vi "LWXPS_GroupMoveAbsolute.vi"(0 "XPS Reference IN":refnum<k24>, 5 "Group Name":string, 7 "Target Position IN":dbl[](array[numeric]), 9 "Number of Positioners":i32, 11 "LabVIEW error IN":errorcluster) -> (4 "XPS Reference OUT":refnum<k24>, 6 "Returned error code":i32, 8 "Target Position OUT":dbl[](array[numeric]), 10 "XPS Error String":string, 15 "LabVIEW error OUT":errorcluster)   [LabVIEW 2020]
uses:
  C:/Users/loasis.BELLANET/Downloads/XPS-UNIFIED/LabVIEW VIs/LabVIEW Source Code/Dll/Newport.XPS.CommandInterface.dll
  Users/loasis.BELLANET/Downloads/XPS-UNIFIED/LabVIEW VIs/LabVIEW Source Code/Dll/Newport.XPS.CommandInterface.dll
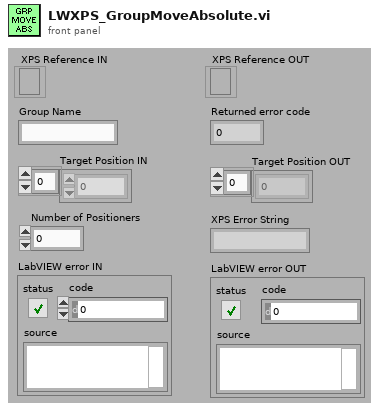
[diagram p1: front panel]
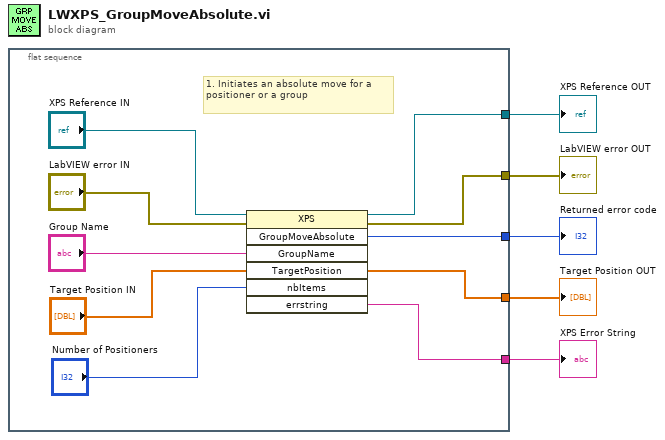
[diagram p0: block diagram]
diagram:
  n1 = flat-sequence {
    tunnel: [w13] -> w5
    tunnel: [w10] -> w4
    tunnel: [w14] -> w3
    tunnel: [w6] -> w2
    tunnel: [w9] -> w1
    frame #0 {
      # "1. Initiates an absolute move for a positioner or a group"
      n2 = invoke class="XPS" method="GroupMoveAbsolute"(reference="XPS Reference IN", error in="LabVIEW error IN", "GroupName"="Group Name", "TargetPosition"="Target Position IN", "nbItems"="Number of Positioners") -> (reference out=w13:refnum<k24>, error out=w10:errorcluster, "GroupMoveAbsolute"=w14:i32, "TargetPosition"=w9:dbl[], "errstring"=w6:string)  [unwired: 2 in, 2 out]
    }
  }
  "XPS Reference OUT" <- w5
  "LabVIEW error OUT" <- w4
  "Returned error code" <- w3
  "XPS Error String" <- w2
  "Target Position OUT" <- w1
